vi "Write Z_Source.vi"(8 "error in (no error)":errorcluster, 10 "Z_Source":T1, 11 "Z_HSw in":refnum<class "Z_HSw.lvclass">) -> (0 "error out":errorcluster, 3 "Z_HSw out":refnum<class "Z_HSw.lvclass">)   [LabVIEW 2019, in "Z_HSw.lvclass"]
uses:
  Z_HSw.lvclass
  Z_source.ctl
  Z_HSw.lvclass/Z_HSw.ctl
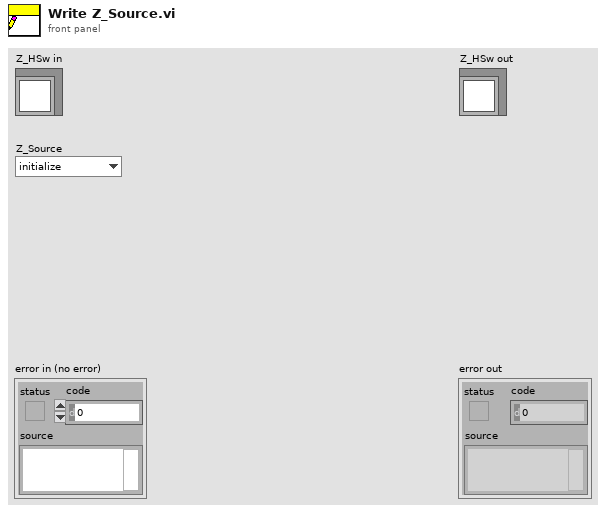
[diagram p1: front panel]
types:
  T1 = typedef "Z_source.ctl" = enum8{"initialize", "local disabled", "local hand", "hand", "auto", "dist"}
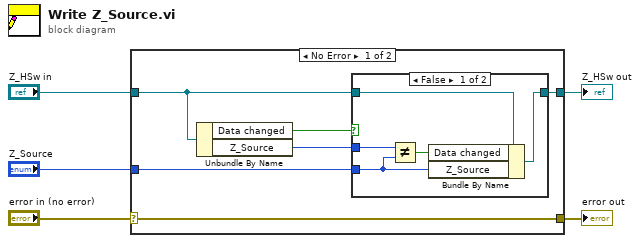
[diagram p0: block diagram]
diagram:
  n1 = case shown="No Error" "error in (no error)" {
    selector: "error in (no error)" -> [w11 w18]
    tunnel: [w11 w18] -> w4
    tunnel: [w10 w19] -> w2
    tunnel: "Z_HSw in" -> [w9 w19]
    tunnel: "Z_Source" -> [w7 _]
    frame No Error {
      n2 = Unbundle By Name(w9) -> ("Data changed"=w6:bool, "Z_Source"=w8:T1)
      n3 = case shown="False" w6 {
        tunnel: [w16 w17] -> w10
        tunnel: w9 -> [w15 w17]
        tunnel: w8 -> [w14 _]
        tunnel: w7 -> [w13 _]
        frame False {
          n4 = Not Equal?(x=w14, y=w13) -> (x != y?=w12:bool)
          n5 = Bundle By Name(cluster=w15, "Data changed"=w12, "Z_Source"=w13) -> (w16:refnum<class "Z_HSw.lvclass">)
        }
        frame True {
        }
      }
    }
    frame Error {
    }
  }
  "error out" <- w4
  "Z_HSw out" <- w2
